vi "Flipper Control.vi"(1 "InFlipper":bool, 2 "FlipperAtPlace":bool, 3 "FrisbiInCannon":bool) -> (0 "Flipper Direction":i32)   [LabVIEW 2012]
panel:
  # "Flipper Directions:\n+1 : up\n0 : don't move\n-1 : down"
  # "Cannon"
  # "InFlipper"
  # "FlipperAtPlace"
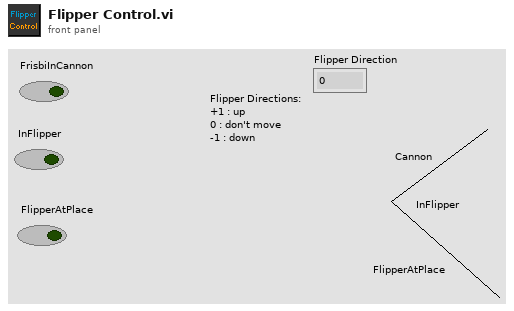
[diagram p1: front panel]
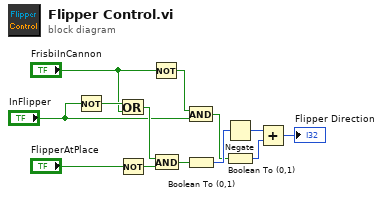
[diagram p0: block diagram]
diagram:
  n1 = Not(x="InFlipper") -> (.not. x?=w10:bool)
  n2 = Or(x=w10, y="FrisbiInCannon") -> (x .or. y?=w11:bool)
  n3 = Not(x="FlipperAtPlace") -> (.not. x?=w12:bool)
  n4 = Not(x="FrisbiInCannon") -> (.not. x?=w6:bool)
  n5 = And(x=w11, y=w12) -> (x .and. y?=w9:bool)
  n6 = And(x=w6, y="InFlipper") -> (x .and. y?=w4:bool)
  n7 = Boolean To (0,1)(Boolean=w9) -> (0, 1=w8:i16)
  n8 = Negate(x=w8) -> (-x=w3:i16)
  n9 = Boolean To (0,1)(Boolean=w4) -> (0, 1=w2:i16)
  n10 = Add(x=w3, y=w2) -> (x+y=→"Flipper Direction":i16)
